vi "PCert-ConfigPageNF-CloseActorConn.vi"(8 "error in (no error)":errorcluster, 11 "ERP-ConfigPageNF in":refnum<class "PCert-ConfigPageNF.lvclass">) -> (0 "error out":errorcluster, 3 "ERP-ConfigPageNF out":refnum<class "PCert-ConfigPageNF.lvclass">)   [LabVIEW 2013, in "PCert-ConfigPageNF.lvclass"]
uses:
  PCert-ConfigPageNF.lvclass
  PCert-ConfigPageNF.lvclass/PCert-ConfigPageNF.ctl
  ftw-dataflow/Actor/src/Connector/FTW-ActorConnector.lvclass
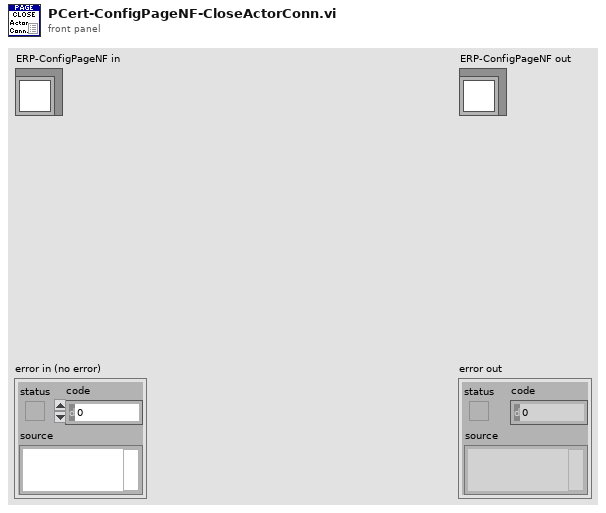
[diagram p1: front panel]
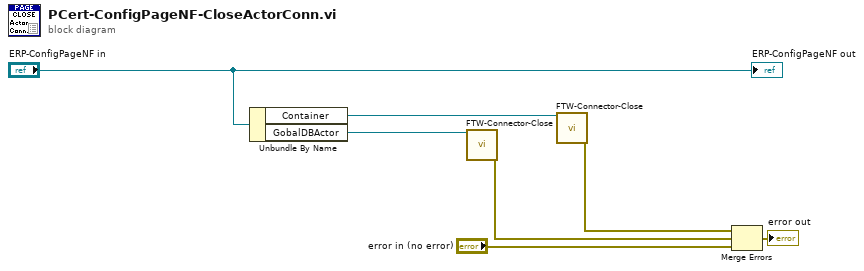
[diagram p0: block diagram]
diagram:
  n1 = Unbundle By Name("ERP-ConfigPageNF in") -> ("Container"=w5:refnum<class "FTW-ActorConnector.lvclass">, "GobalDBActor"=w6:refnum<class "FTW-ActorConnector.lvclass">)
  n2 = call-dynamic "FTW-Connector-Close.vi"("FTW Actor Connector"=w6) -> ("error out"=w3:errorcluster)  [unwired: 14 in]
  n3 = call-dynamic "FTW-Connector-Close.vi"("FTW Actor Connector"=w5) -> ("error out"=w2:errorcluster)  [unwired: 14 in]
  n4 = Merge Errors(w2, w3, "error in (no error)") -> (→"error out":errorcluster)
  "ERP-ConfigPageNF out" <- "ERP-ConfigPageNF in"
